vi "SetValueByHierarchicalPathArray.vi"(0 "VI Reference In":refnum<vi>, 2 "delimiter (>>)":string=">>", 5 "Control Path":string, 7 "Hierarchical Path Array":string[](array[string]), 11 "Error In":errorcluster) -> (4 "VI Reference Out":refnum<vi>, 15 "Error Out":errorcluster)   [LabVIEW 2016, in "Drona.lvlib" / "ControlValue.lvlib" / "StimulusTree.lvlib"]
doc: "Sets value(signaling) for the multi-select tree control whose hierarchical path for each items are specified as an array. \n\nHierarchical path represent their corresponding parents of an item from its origin. Use the delimiters '>>' between each hierarchy in the path\n\nFor example to select the item 'Child3', give the hierarchical path as \"<b>Parent1</b>(top level parent in tree)<b>>>Child1</b>(children for parent1)<b>>>Child2</b>(children for child1)<b>>>Child3</b>(children for child2)\"\n\nThe input control name is given as a string , incase of path, use delimiters inbetween the path."
uses:
  StimulusTree.lvlib
  <vilib>/Utility/error.llb/Error Cluster From Error Code.vi
  <vilib>/ErrorRing/Error Ring.xnode
  Drona.lvlib
  Get/GetControlRef/GetControlRef.lvlib
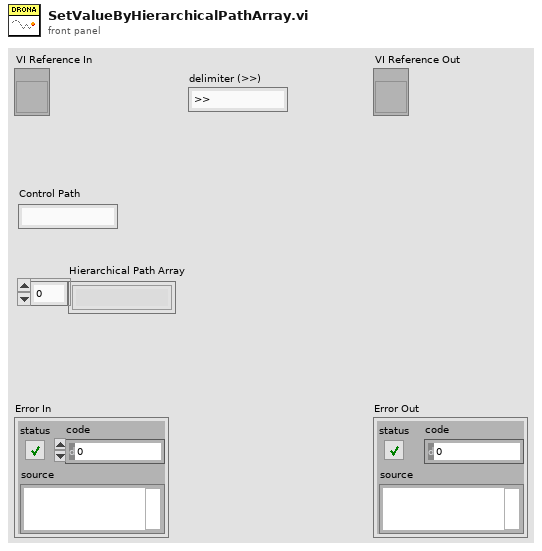
[diagram p1: front panel]
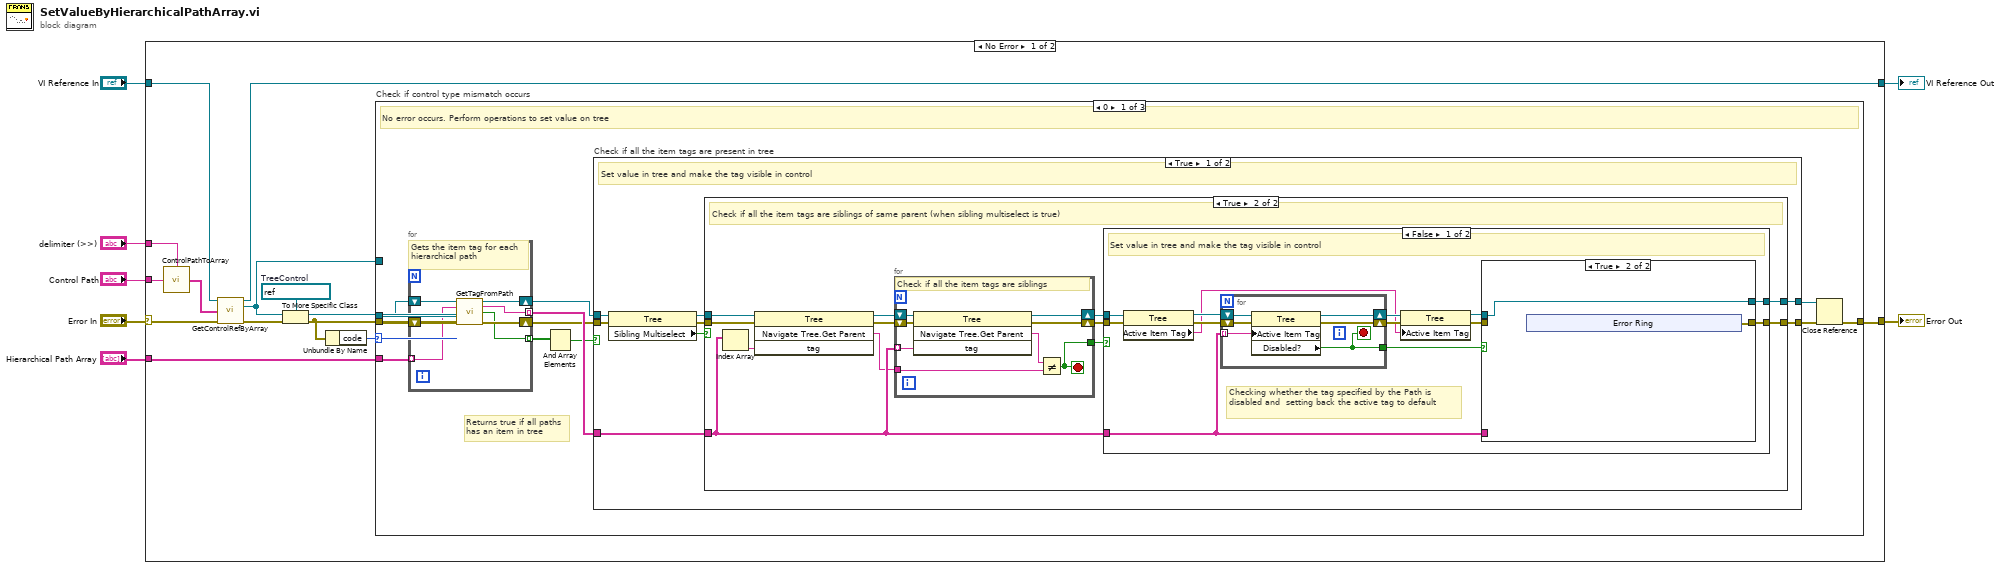
[diagram p0: block diagram]
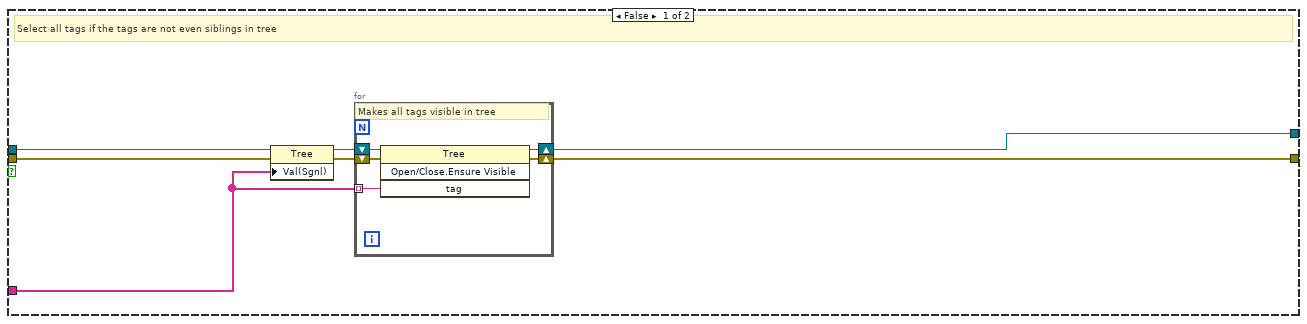
[diagram p2: hidden frame]
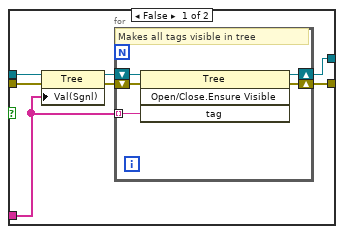
[diagram p3: hidden frame]
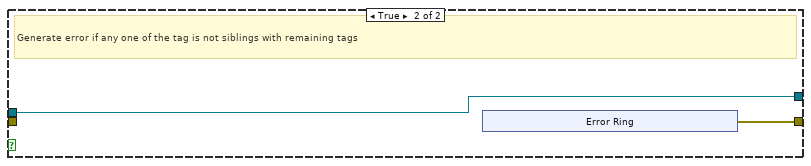
[diagram p4: hidden frame]
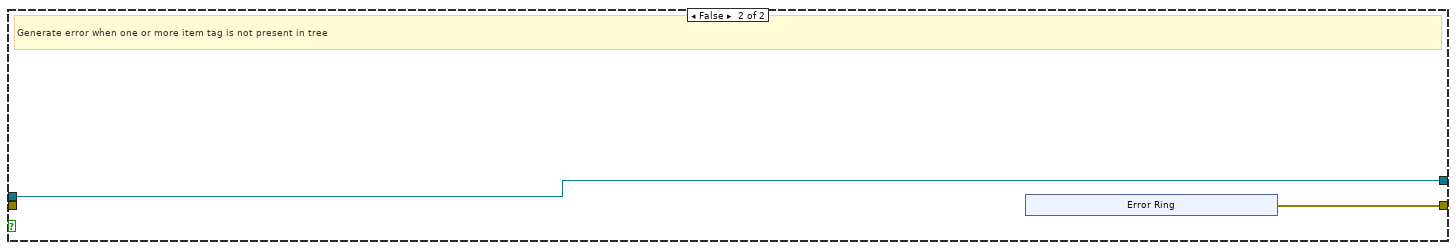
[diagram p5: hidden frame]
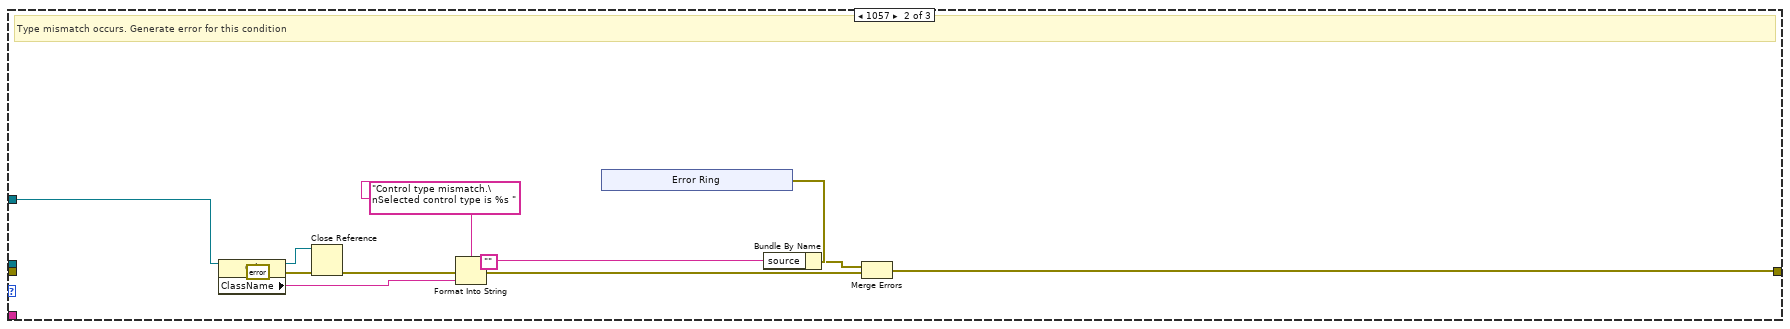
[diagram p6: hidden frame]
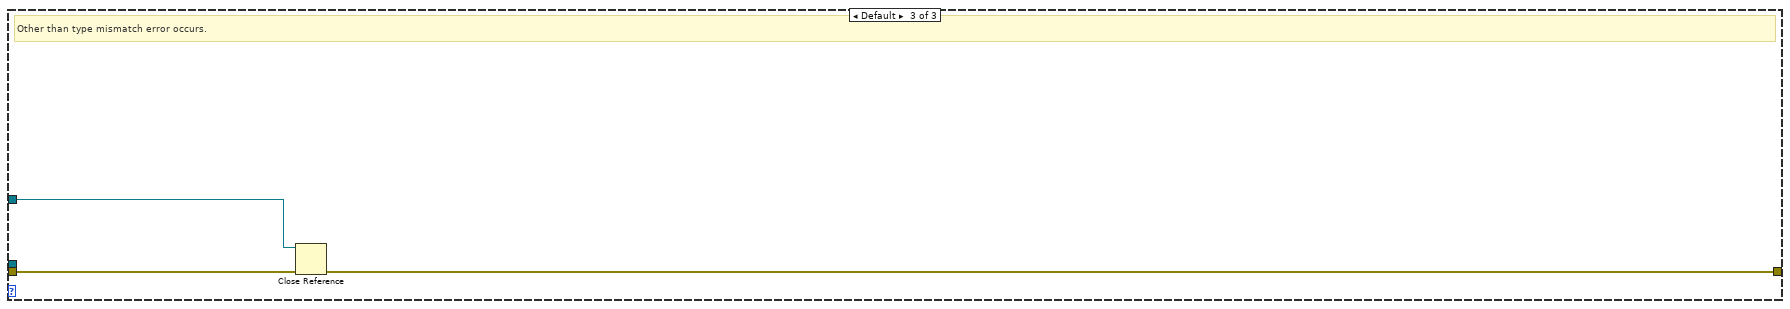
[diagram p7: hidden frame]
diagram:
  n1 = case shown="No Error" "Error In" {
    selector: "Error In" -> [w18 w154]
    tunnel: [w9 w154] -> w6
    tunnel: "VI Reference In" -> [w17 w153]
    tunnel: "Control Path" -> [w20 _]
    tunnel: [w14 w153] -> w3
    tunnel: "delimiter (>>)" -> [w19 _]
    tunnel: "Hierarchical Path Array" -> [w8 _]
    frame No Error {
      w21 = refnum<vi> refnum  # TreeControl
      n2 = call "ControlPathToArray.vi"("Control Name"=w20, "delimiter (>>)"=w19) -> ("Control Path"=w16:string[])
      n3 = call "GetControlRefByArray.vi"("VI Reference In"=w17, "Control Path"=w16, "error In"=w18) -> ("VI Reference Out"=w14:refnum<vi>, "Ctl Refnum"=w11:refnum<vi>, "error out"=w15:errorcluster)  [unwired: 10 in]
      n4 = To More Specific Class(target class=w21, reference=w11, error in=w15) -> (specific class reference=w12:refnum<vi>, error out=w13:errorcluster)
      n5 = Unbundle By Name(w13) -> ("code"=w10:i32)
      n6 = case "Check if control type mismatch occurs" shown="0" w10 {
        tunnel: [w23 w135 w151] -> w9
        tunnel: w12 -> [w31 _ _]
        tunnel: w8 -> [w32 _ _]
        tunnel: w11 -> [_ w144 w150]
        tunnel: w13 -> [w30 _ w152]
        frame 0 {
          # "Returns true if all paths\nhas an item in tree"
          # "No error occurs. Perform operations to set value on tree"
          n7 = for {
            tunnel: w32 -> [w128] mode=indexing
            tunnel: [w127] -> w28 mode=indexing
            shift-right: [w126] -> w25
            shift-left: w31 -> [w129]
            shift-right: [w130] -> w26
            shift-left: w30 -> [w131]
            tunnel: [w125] -> w29 mode=indexing
            # "Gets the item tag for each hierarchical path"
            n8 = call "GetTagFromPath.vi"("Tree Ref In"=w129, "Hierarchical Path"=w128, "Error In"=w131) -> ("Tree Ref Out"=w126:refnum<vi>, "Item Tag"=w127:string, "Item Found?"=w125:bool, "Error Out"=w130:errorcluster)  [unwired: 9 in]
          }
          n9 = And Array Elements(Boolean array=w29) -> (logical AND=w27:bool)
          n10 = case "Check if all the item tags are present in tree" shown="True" w27 {
            tunnel: [w39 w118] -> w24
            tunnel: [w38 w119] -> w22
            tunnel: w26 -> [w40 _]
            tunnel: w25 -> [w35 w119]
            tunnel: w28 -> [w37 _]
            frame True {
              # "Set value in tree and make the tag visible in control"
              n11 = property class="Tree"(reference=w35, error in=w40) -> (reference out=w33:refnum<vi>, error out=w36:errorcluster, "Sibling Multiselect"=w34:bool)
              n12 = case shown="True" w34 {
                tunnel: [w46 w64] -> w39
                tunnel: [w44 w63] -> w38
                tunnel: w37 -> [w43 w59]
                tunnel: w36 -> [w42 w62]
                tunnel: w33 -> [w41 w60]
                frame False {
                  # "Select all tags if the tags are not even siblings in tree"
                  n13 = property class="Tree"(reference=w41, error in=w42, "Val(Sgnl)"=w43) -> (reference out=w45:refnum<vi>, error out=w47:errorcluster)
                  n14 = for {
                    shift-right: [w51] -> w46
                    shift-left: w47 -> [w52]
                    shift-right: [w49] -> w44
                    shift-left: w45 -> [w50]
                    tunnel: w43 -> [w48] mode=indexing
                    # "Makes all tags visible in tree"
                    n15 = invoke class="Tree" method="Open/Close.Ensure Visible"(reference=w50, error in=w52, "tag"=w48) -> (reference out=w49:refnum<vi>, error out=w51:errorcluster)  [unwired: 1 in, 2 out]
                  }
                }
                frame True {
                  # "Check if all the item tags are siblings of same parent (when sibling multiselect is true)"
                  n16 = Index Array(array=w59) -> (element=w58:string)  [unwired: 1 in]
                  n17 = invoke class="Tree" method="Navigate Tree.Get Parent"(reference=w60, error in=w62, "tag"=w58) -> (reference out=w53:refnum<vi>, error out=w61:errorcluster, "Navigate Tree:Get Parent"=w57:string)  [unwired: 1 in, 1 out]
                  n18 = for {
                    tunnel: w59 -> [w115] mode=indexing
                    shift-right: [w113] -> w55
                    shift-left: w61 -> [w116]
                    shift-right: [w114] -> w54
                    shift-left: w53 -> [w117]
                    tunnel: w57 -> [w111]
                    tunnel: [w110] -> w56
                    stop <- w110 stop-if-true
                    # "Check if all the item tags are siblings"
                    n19 = invoke class="Tree" method="Navigate Tree.Get Parent"(reference=w117, error in=w116, "tag"=w115) -> (reference out=w114:refnum<vi>, error out=w113:errorcluster, "Navigate Tree:Get Parent"=w112:string)  [unwired: 1 in, 1 out]
                    n20 = Not Equal?(x=w112, y=w111) -> (x != y?=w110:bool)
                  }
                  n21 = case shown="False" w56 {
                    tunnel: [w77 w103] -> w64
                    tunnel: [w76 w104] -> w63
                    tunnel: w59 -> [w66 _]
                    tunnel: w55 -> [w69 _]
                    tunnel: w54 -> [w70 w104]
                    frame False {
                      # "Checking whether the tag specified by the Path is disabled and  setting back the active tag to default"
                      # "Set value in tree and make the tag visible in control"
                      n22 = property class="Tree"(reference=w70, error in=w69) -> (reference out=w72:refnum<vi>, error out=w73:errorcluster, "Active Item Tag"=w71:string)
                      n23 = for {
                        tunnel: w66 -> [w83] mode=indexing
                        tunnel: [w82] -> w65
                        shift-right: [w81] -> w74
                        shift-left: w73 -> [w80]
                        shift-right: [w79] -> w75
                        shift-left: w72 -> [w78]
                        stop <- w82 stop-if-true
                        n24 = property class="Tree"(reference=w78, error in=w80, "Active Item Tag"=w83) -> (reference out=w79:refnum<vi>, error out=w81:errorcluster, "Disabled?"=w82:bool)
                      }
                      n25 = property class="Tree"(reference=w75, error in=w74, "Active Item Tag"=w71) -> (reference out=w68:refnum<vi>, error out=w67:errorcluster)
                      n26 = case shown="True" w65 {
                        tunnel: [w89 w97] -> w77
                        tunnel: [w87 w96] -> w76
                        tunnel: w66 -> [w86 _]
                        tunnel: w67 -> [w85 _]
                        tunnel: w68 -> [w84 w96]
                        frame False {
                          n27 = property class="Tree"(reference=w84, error in=w85, "Val(Sgnl)"=w86) -> (reference out=w88:refnum<vi>, error out=w90:errorcluster)
                          n28 = for {
                            shift-right: [w94] -> w89
                            shift-left: w90 -> [w95]
                            shift-right: [w92] -> w87
                            shift-left: w88 -> [w93]
                            tunnel: w86 -> [w91] mode=indexing
                            # "Makes all tags visible in tree"
                            n29 = invoke class="Tree" method="Open/Close.Ensure Visible"(reference=w93, error in=w95, "tag"=w91) -> (reference out=w92:refnum<vi>, error out=w94:errorcluster)  [unwired: 1 in, 2 out]
                          }
                        }
                        frame True {
                          n30 = xnode "Error Ring"() -> ("error out"=w97:errorcluster)
                        }
                      }
                    }
                    frame True {
                      # "Generate error if any one of the tag is not siblings with remaining tags"
                      n31 = xnode "Error Ring"() -> ("error out"=w103:errorcluster)
                    }
                  }
                }
              }
            }
            frame False {
              # "Generate error when one or more item tag is not present in tree"
              n32 = xnode "Error Ring"() -> ("error out"=w118:errorcluster)
            }
          }
          n33 = Close Reference(reference=w22, error in (no error)=w24) -> (error out=w23:errorcluster)
        }
        frame 1057 {
          # "Type mismatch occurs. Generate error for this condition"
          n34 = property class="Ctl"(reference=w144, error in=errorcluster {"status"=FALSE, "code"=0, "source"=""} ("error out")) -> (reference out=w133:refnum<vi>, error out=w143:errorcluster, "ClassName"=w141:string)
          n35 = Close Reference(reference=w133, error in (no error)=w143) -> (error out=w134:errorcluster)
          n36 = Format Into String(format string="Control type mismatch.\nSelected control type is %s ", initial string="", error in=w134, w141) -> (resulting string=w138:string, error out=w136:errorcluster)
          n37 = xnode "Error Ring"() -> ("error out"=w139:errorcluster)
          n38 = Bundle By Name(cluster=w139, "source"=w138) -> (w137:errorcluster)
          n39 = Merge Errors(w137, w136) -> (w135:errorcluster)
        }
        frame Default {
          # "Other than type mismatch error occurs."
          n40 = Close Reference(reference=w150, error in (no error)=w152) -> (error out=w151:errorcluster)
        }
      }
    }
    frame Error {
    }
  }
  "Error Out" <- w6
  "VI Reference Out" <- w3
